vi "mro get Negative Coils Lock Intensity(not implemented).vi"(8 "error in (no error)":errorcluster, 10 "status":i32, 11 "val":dbl) -> (0 "error out":errorcluster, 1 "function return":i8, 2 "status out":i32, 3 "val out":dbl)   [LabVIEW 2016]
doc: "MIRAOEXPORT MroBoolean MIRAOCALL mro_getNegativeCoilsLockIntensity(\n MroIntensity* val,\n int* status\n );"
uses:
  mirao52e.dll
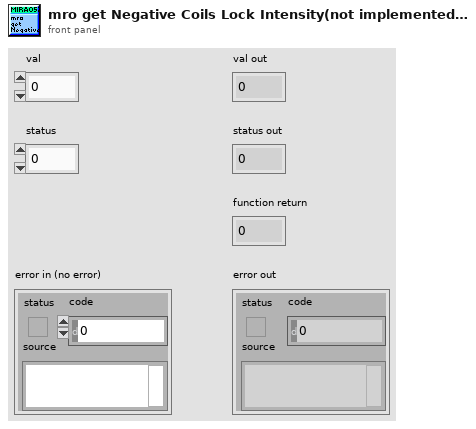
[diagram p1: front panel]
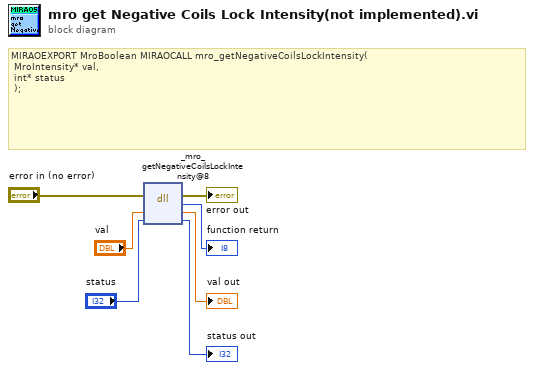
[diagram p0: block diagram]
diagram:
  # "MIRAOEXPORT MroBoolean MIRAOCALL mro_getNegativeCoilsLockIntensity(\n\tMroIntensity* val,\n\tint* status\n\t);"
  n1 = dll-call lib="C:/Users/nvladim/Documents/Nikita-MDC/code/LabView/miraoDriver_32bit/mirao52e.*" fn="_mro_getNegativeCoilsLockIntensity@8"(error in="error in (no error)", "val"="val", "status"="status") -> (error out=→"error out":errorcluster, →"function return":i8, "val"=→"val out":dbl, "status"=→"status out":i32)  [unwired: 2 in, 1 out]
